vi "set test state（三态）.vi"(2 "Timeout in":u32=1000, 4 "启动(T启动\\F停止)":bool, 6 "error in":errorcluster, 7 "Slave Address":u8=255, 8 "启动单次":bool, 9 "VISA resource name in":refnum<visa-resource-name>="COM1") -> (0 "error out":errorcluster, 1 "Serial Parameters":T1, 3 "VISA resource name out":refnum<visa-resource-name>, 5 "Timeout out":u32=1000)   [LabVIEW 2018]
uses:
  NI Modbus.llb/MB Serial Master Query Write Single Register (poly).vi
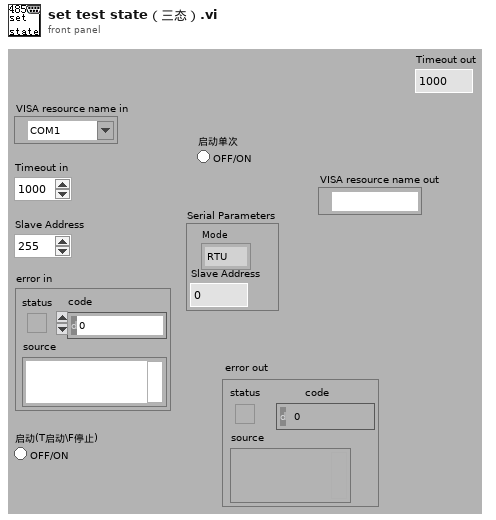
[diagram p1: front panel]
types:
  T1 = cluster{"Mode":enum16{"RTU", "ASCII"}, "Slave Address":u8}
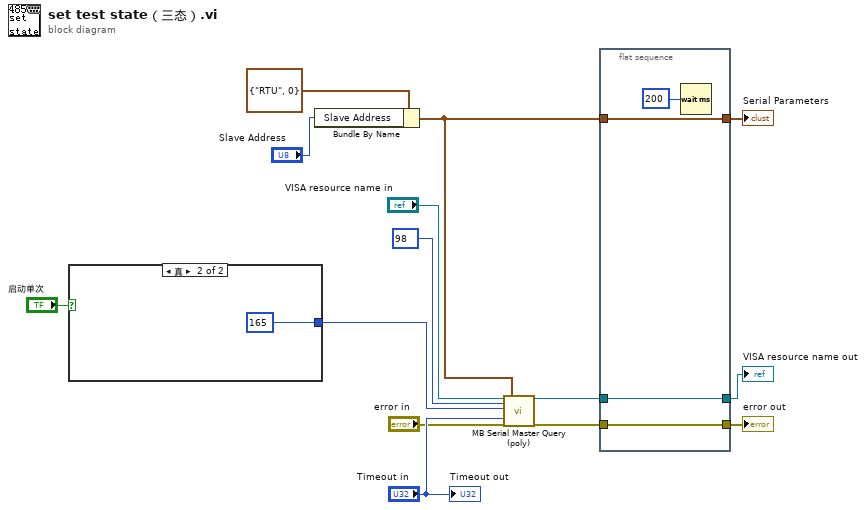
[diagram p0: block diagram]
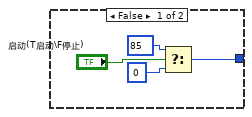
[diagram p2: hidden frame]
diagram:
  n1 = case shown="真" "启动单次" {
    tunnel: [w15 u16 165 ("Holding Register")] -> w2
    frame False {
      n2 = Select(t=u16 85 ("Holding Register"), s="启动(T启动\\F停止)", f=u16 0 ("Holding Register")) -> (s? t:f=w15:u16)
    }
    frame True {
    }
  }
  n3 = Bundle By Name(cluster=T1 {"Mode"=enum."RTU", "Slave Address"=0} ("Serial Parameters"), "Slave Address"="Slave Address") -> (w11:T1)
  n4 = call-poly "MB Serial Master Query (poly).vi"("VISA resource name"="VISA resource name in", "Address"=u16 98, "Holding Register"=w2, "Timeout"="Timeout in", "error in"="error in", "Serial Parameters"=w11) -> ("VISA resource name out"=w4:refnum<visa-resource-name>, "error out"=w3:errorcluster)  [unwired: 11 in, 1 out]
  n5 = flat-sequence {
    tunnel: [w23] -> w10
    tunnel: w4 -> [w23]
    tunnel: [w22] -> w12
    tunnel: w11 -> [w22]
    tunnel: [w21] -> w6
    tunnel: w3 -> [w21]
    frame #0 {
      n6 = Wait (ms)(milliseconds to wait=u32 200) -> ()  [unwired: 1 out]
    }
  }
  "error out" <- w6
  "Serial Parameters" <- w12
  "VISA resource name out" <- w10
  "Timeout out" <- "Timeout in"
